vi "PH_GetBBInformation.get and prepare Info.vi"(5 "error in":errorcluster) -> (14 "ColHdrs[]":string[](array[string])=["Sixpack Instance", "Axis"], 15 "RowHdrs[]":string[](array[string]), 16 "ItemNames":string[][](array[string]), 17 "Row Cell BG":u32[](array[numeric]), 19 "error out":errorcluster)   [LabVIEW 2014, in "PH_GetBBInformation.lvlib"]
doc: "This VI is reading out information from the database and prepares it for the visualisation on the GUI."
uses:
  PH_GetBBInformation.lvlib
  PH_Common/PH_Common.lvlib
  CSCore/CSSystem/CSSystemLib/CSSystemLib.lvlib
  PH_PSDBWriter/PH_PSDBWriter.lvlib
  PH_BlackBox/PH_BlackBox.lvlib
  PH_Beckhoff_Common/PH_Beckhoff_Common.lvlib
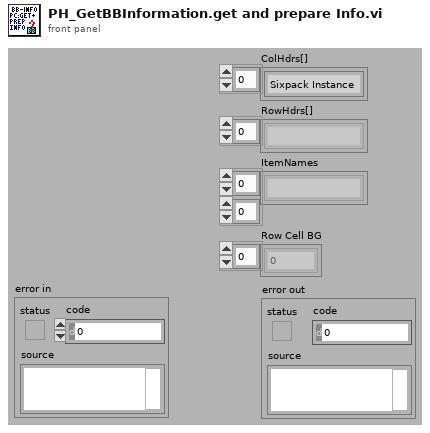
[diagram p1: front panel]
types:
  T1 = typedef "PH_Beckhoff_Common.lvlib/PH_Beckhoff_Common.BB Tagnames.ctl" = cluster{"Sensor Remote controlled":string, "Sensor Out":string, "Sensor In":string, "Actor Direction In":string, "Actor Move":string, "Sensor Power ok":string, "Instance":string}
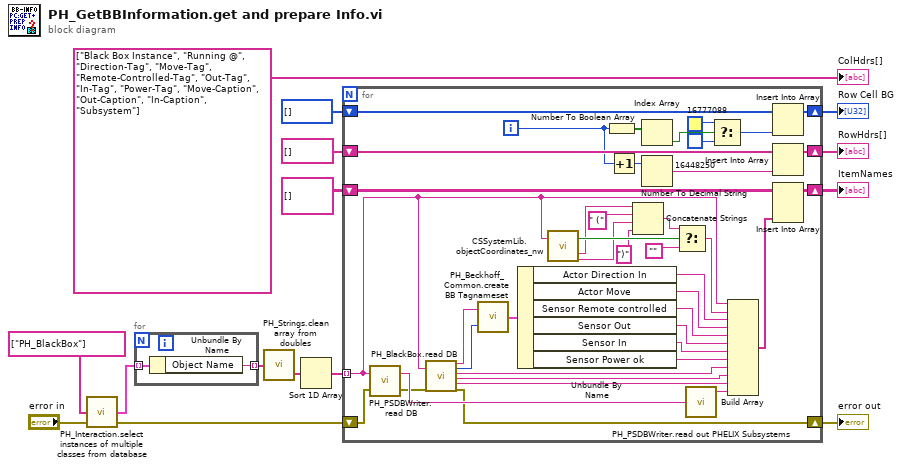
[diagram p0: block diagram]
diagram:
  n1 = call "PH_Interaction.select instances of multiple classes from database.vi"("error in (no error)"="error in", "Classes Input"=string[] ["PH_BlackBox"]) -> ("error out"=w5:errorcluster, "Query Result"=w4:cluster{"Object Name":string, "Class":string}[])  [unwired: 2 in]
  n2 = for {
    tunnel: w4 -> [w17] mode=indexing
    tunnel: [w16] -> w3 mode=indexing
    n3 = Unbundle By Name(w17) -> ("Object Name"=w16:string)
  }
  n4 = call "PH_Strings.clean array from doubles.vi"("Array Input"=w3) -> ("Cleaned Array Output"=w2:string[])  [unwired: 1 out]
  n5 = Sort 1D Array(array=w2) -> (sorted array=w1:string[])
  n6 = for {
    tunnel: w1 -> [w18] mode=indexing
    shift-right: [w58] -> w10
    shift-left: string[][] [] -> [w57]
    shift-right: [w54] -> w12
    shift-left: string[] [] -> [w55]
    shift-right: [w52] -> w14
    shift-left: u32[] [] -> [w51]
    shift-right: [w19] -> w15
    shift-left: w5 -> [w20]
    i -> [w42]
    n7 = call "PH_PSDBWriter.read DB.vi"("error in"=w20, "Instance Name"=w18) -> ("error out"=w21:errorcluster, "PSDB Subsystem"=w35:string)
    n8 = call "PH_BlackBox.read DB.vi"("BB Instance"=w18, "error in (no error)"=w21) -> ("Recipient"=w31:string, "#"=w30:i32, "Caption Move"=w32:string, "Caption Out"=w33:string, "Caption In"=w34:string, "error out"=w19:errorcluster)  [unwired: 12 in]
    n9 = call "PH_Beckhoff_Common.create BB Tagnameset.vi"("#"=w30, "Instance Name"=w31) -> ("output cluster"=w29:T1)
    n10 = Unbundle By Name(w29) -> ("Actor Direction In"=w28:string, "Actor Move"=w27:string, "Sensor Remote controlled"=w26:string, "Sensor Out"=w25:string, "Sensor In"=w24:string, "Sensor Power ok"=w23:string)
    n11 = call "CSSystemLib.objectCoordinates_nw.vi"("name"=w18) -> ("obj exists"=w50:bool, "systemID"=w48:string, "node"=w45:string)  [unwired: 15 in, 1 out]
    n12 = Number To Boolean Array(number=w42) -> (Boolean array=w39:bool[])
    n13 = Increment(x=w42) -> (x+1=w41:i32)
    n14 = Concatenate Strings(w48, " (" ("string"), w45, ")" ("string")) -> (w47:string)
    n15 = Index Array(array=w39) -> (element=w40:bool)  [unwired: 1 in]
    n16 = Number To Decimal String(number=w41) -> (decimal integer string=w56:string)  [unwired: 1 in]
    n17 = Select(t=w47, s=w50, f="") -> (s? t:f=w22:string)
    n18 = call "PH_PSDBWriter.read out PHELIX Subsystems.vi"("Config DB Subsystem"=w35) -> ("Subsystem"=w36:string)  [unwired: 2 in, 2 out]
    n19 = Select(t=u32 16777088 ("Color Box"), s=w40, f=u32 16448250 ("Color Box")) -> (s? t:f=w53:u32)
    n20 = Build Array(w18, w22, w28, w27, w26, w25, w24, w23, w32, w33, w34, w36) -> (w43:string[])
    n21 = Insert Into Array(array=w51, new element=w53) -> (w52:u32[])  [unwired: 1 in]
    n22 = Insert Into Array(array=w55, new element=w56) -> (w54:string[])  [unwired: 1 in]
    n23 = Insert Into Array(array=w57, new element=w43) -> (w58:string[][])  [unwired: 2 in]
  }
  "error out" <- w15
  "Row Cell BG" <- w14
  "RowHdrs[]" <- w12
  "ItemNames" <- w10
  "ColHdrs[]" <- string[] ["Black Box Instance", "Running @", "Direction-Tag", "Move-Tag", "Remote-Controlled-Tag", "Out-Tag", "In-Tag", "Power-Tag", "Move-Caption", "Out-Caption", "In-Caption", "Subsystem"] ("new element/subarray")
